vi "Numbers to Colors.vi"(1 "Left Stim Pattern Values":T1[][](array[typedef])) -> (0 "Stim Pattern Array":u32[][](array[colorbox]))   [LabVIEW 2019]
uses:
  Stim off-half-ful.ctl
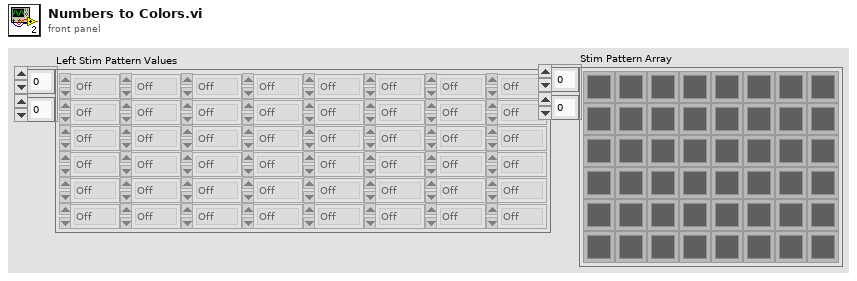
[diagram p1: front panel]
types:
  T1 = typedef "Stim off-half-ful.ctl" = enum16{"Off", "Half", "Full"}
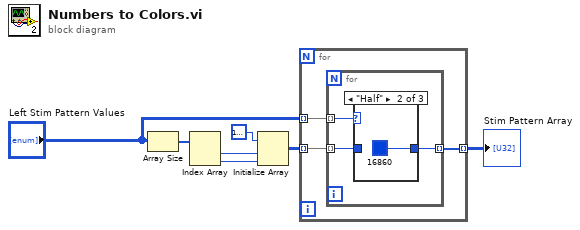
[diagram p0: block diagram]
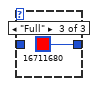
[diagram p3: hidden frame]
diagram:
  n1 = Array Size(array="Left Stim Pattern Values") -> (size(s)=w6:i32[])
  n2 = Index Array(array=w6) -> (element #1=w5:i32, element #2=w4:i32)  [unwired: 2 in]
  n3 = Initialize Array(u32 16777222 ("Color Box"), w5, w4) -> (w2:u32[][])
  n4 = for {
    tunnel: "Left Stim Pattern Values" -> [w10] mode=indexing
    tunnel: w2 -> [w9] mode=indexing
    tunnel: [w8] -> w1 mode=indexing
    n5 = for {
      tunnel: w10 -> [w13] mode=indexing
      tunnel: w9 -> [w12] mode=indexing
      tunnel: [w11] -> w8 mode=indexing
      n6 = case shown="\"Half\"" w13 {
        tunnel: w12 -> [w14 _ _]
        tunnel: [w14 u32 16860 ("Color Box") u32 16711680 ("Color Box")] -> w11
        frame "Off", Default {
        }
        frame "Half" {
        }
        frame "Full" {
        }
      }
    }
  }
  "Stim Pattern Array" <- w1
